vi "ReadWorkspaceManager.vi"(8 "error in (no error)":errorcluster, 11 "VeriStand Test Case in":refnum<class "VeriStandTestCase.lvclass">) -> (0 "error out":errorcluster, 2 "Workspace":T1, 3 "VeriStand Test Case out":refnum<class "VeriStandTestCase.lvclass">)   [LabVIEW 2016, in "VeriStandTestCase.lvclass"]
uses:
  VeriStandTestCase.lvclass
  <vilib>/NI Veristand/Execution/Workspace/WorkspaceAPI.ctl
  NationalInstruments.VeriStand.ClientAPI
  VeriStandTestCase.lvclass/VeriStandTestCase.ctl
  <vilib>/NI VeriStand/Execution/Workspace/NI_VS Workspace ExecutionAPI.lvlib
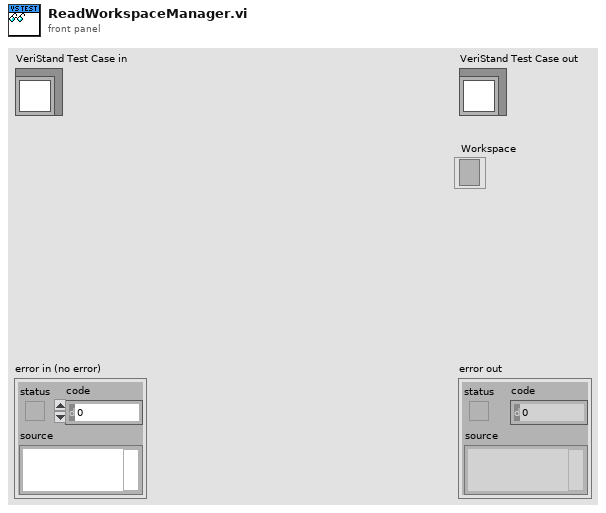
[diagram p1: front panel]
types:
  T1 = typedef "NI_VS Workspace ExecutionAPI.lvlib/WorkspaceAPI.ctl" = refnum<k24>
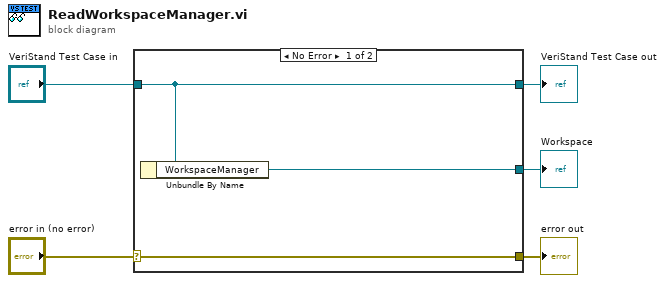
[diagram p0: block diagram]
diagram:
  n1 = case shown="No Error" "error in (no error)" {
    selector: "error in (no error)" -> [w8 w9]
    tunnel: [w8 w9] -> w4
    tunnel: [w7 w10] -> w2
    tunnel: "VeriStand Test Case in" -> [w7 w10]
    tunnel: [w6 _] -> w1
    frame No Error {
      n2 = Unbundle By Name(w7) -> ("WorkspaceManager"=w6:T1)
    }
    frame Error {
    }
  }
  "error out" <- w4
  "VeriStand Test Case out" <- w2
  "Workspace" <- w1
